vi "Transform.vi"(7 "Type X":T1(ring), 8 "error in (no error)":errorcluster caption="entrée d'erreur (pas d'erreur)", 9 "y":string[][](array[string]), 10 "X":string[][](array[string]), 11 "SparseRandomProjection.lvclass":refnum<class "SparseRandomProjection.lvclass">) -> (0 "error out":errorcluster caption="sortie d'erreur", 3 "SparseRandomProjection.lvclass":refnum<class "SparseRandomProjection.lvclass">)   [LabVIEW 2020, in "SparseRandomProjection.lvclass"]
doc: "Project the data by using matrix product with the random matrix\n\nReturns : \n\n- X_new : numpy array or scipy sparse of shape [n_samples, n_components]\nProjected array."
uses:
  SparseRandomProjection.lvclass
  SparseRandomProjection.lvclass/SparseRandomProjection.ctl
panel:
  out "Data":T2
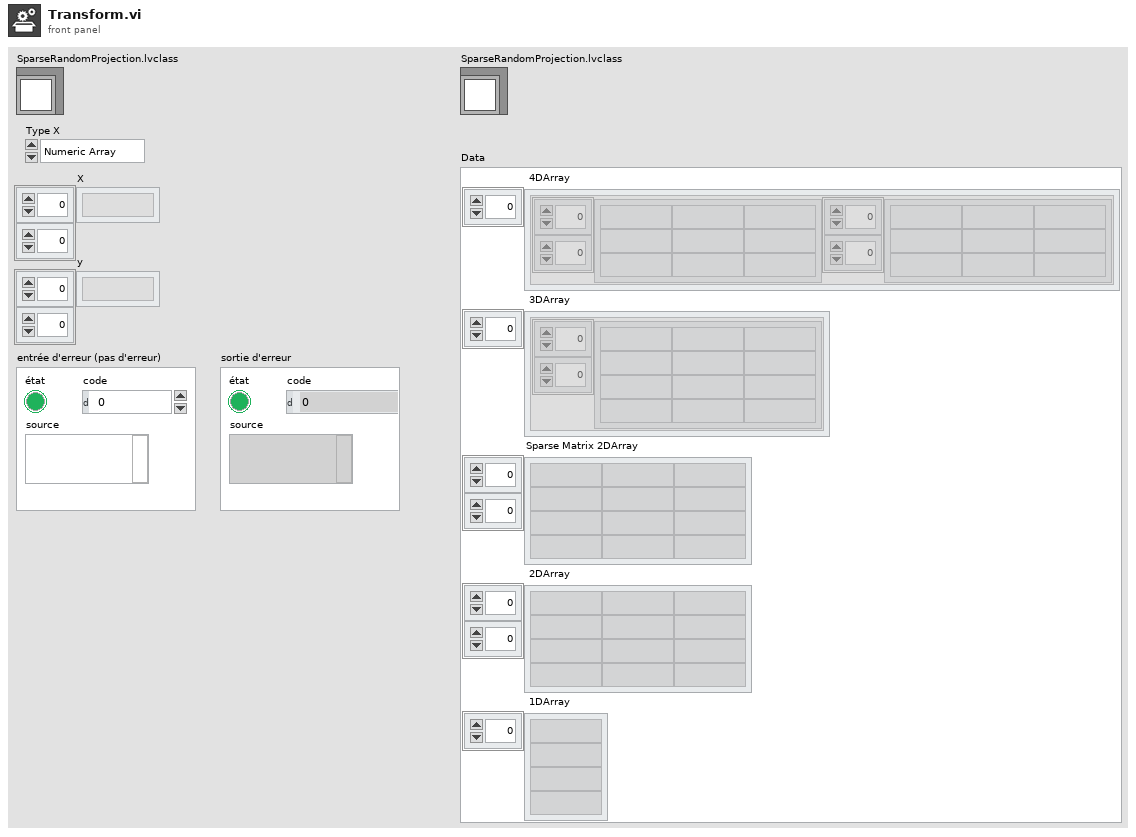
[diagram p1: front panel]
types:
  T1 = enum16{"Numeric Array", "String Array", "Sparse"}
  T2 = cluster{" 4DArray":cluster{"1":string[][], "2":string[][]}[], " 3DArray":cluster{"Tableau":string[][]}[], "Sparse Matrix 2DArray":string[][], " 2DArray":string[][], " 1DArray":string[]}
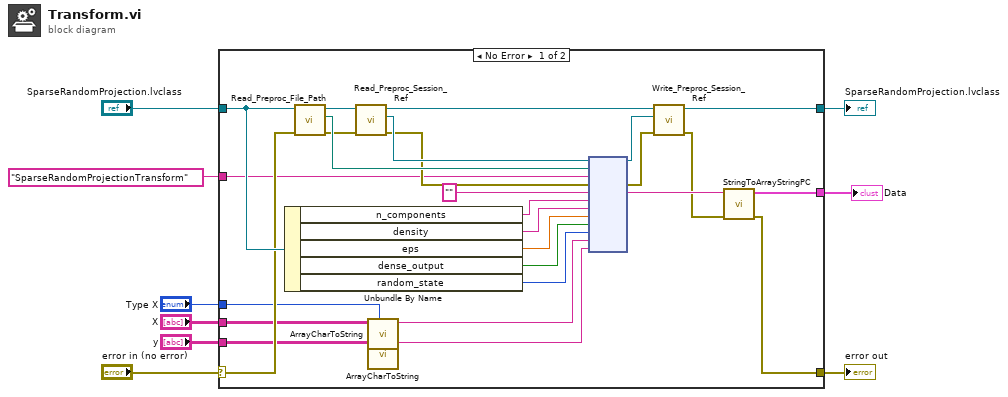
[diagram p0: block diagram]
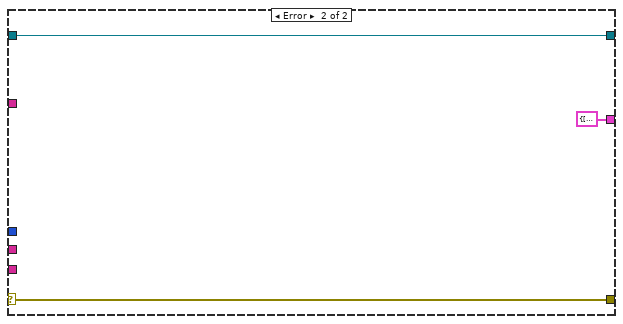
[diagram p2: hidden frame]
diagram:
  n1 = case shown="No Error" "error in (no error)" {
    selector: "error in (no error)" -> [w26 w39]
    tunnel: [w15 w39] -> w8
    tunnel: [w19 w38] -> w6
    tunnel: "SparseRandomProjection.lvclass" -> [w27 w38]
    tunnel: "SparseRandomProjectionTransform" ("Fonction") -> [w25 _]
    tunnel: "X" -> [w14 _]
    tunnel: "y" -> [w12 _]
    tunnel: [w16 T2 {" 4DArray"=[], " 3DArray"=[], "Sparse Matrix 2DArray"=[], " 2DArray"=[], " 1DArray"=[]} ("Data")] -> w2
    tunnel: "Type X" -> [w10 _]
    frame No Error {
      n2 = Unbundle By Name(w27) -> ("n_components"=w24:string, "density"=w23:string, "eps"=w22:dbl, "dense_output"=w21:bool, "random_state"=w20:i32)
      n3 = call-dynamic "Read_Preproc_File_Path.vi"("error in (no error)"=w26, "Python in"=w27) -> ("error out"=w31:errorcluster, "File_Path"=w34:path, "Python out"=w36:refnum<class "SparseRandomProjection.lvclass">)  [unwired: 7 in]
      n4 = call-dynamic "Read_Preproc_Session_Ref.vi"("error in (no error)"=w31, "Python in"=w36) -> ("error out"=w32:errorcluster, "Session_ref"=w33:refnum<k35>, "Python out"=w35:refnum<class "SparseRandomProjection.lvclass">)  [unwired: 7 in]
      n5 = call "ArrayCharToString.vi"("Type"=w10, "TAB"=w14) -> ("Instruction"=w13:string)  [unwired: 9 in]
      n6 = call "ArrayCharToString.vi"("TAB"=w12) -> ("Instruction"=w11:string)  [unwired: 10 in]
      n7 = node(w33, w34, w25, w32, "", w24, w23, w22, w21, w20, w13, w11) -> (w28:refnum<k35>, w30:errorcluster, w18:string)  [unwired: 7 in, 2 out]
      n8 = call-dynamic "Write_Preproc_Session_Ref.vi"("error in (no error)"=w30, "Session_ref"=w28, "Python in"=w35) -> ("error out"=w17:errorcluster, "Python out"=w19:refnum<class "SparseRandomProjection.lvclass">)  [unwired: 7 in]
      n9 = call "StringToArrayStringPC.vi"("sortie d'erreur"=w17, "Return value"=w18) -> ("sortie d'erreur"=w15:errorcluster, "Data"=w16:T2)  [unwired: 8 in]
    }
    frame Error {
    }
  }
  "error out" <- w8
  "SparseRandomProjection.lvclass" <- w6
  "Data" <- w2
